vi "Manip5.vi"() -> ()   [LabVIEW 2021]
uses:
  <vilib>/numeric/Random Number (Range) U64.vi
  <vilib>/numeric/sub_Random U32.vi
panel:
  out "x > 7?":bool
  in  "Delay":u32
  out "Frequence":dbl
  out "Amplitude":dbl
  in  "stop":bool
  out "Waveform Chart":dynamicdata(graph)
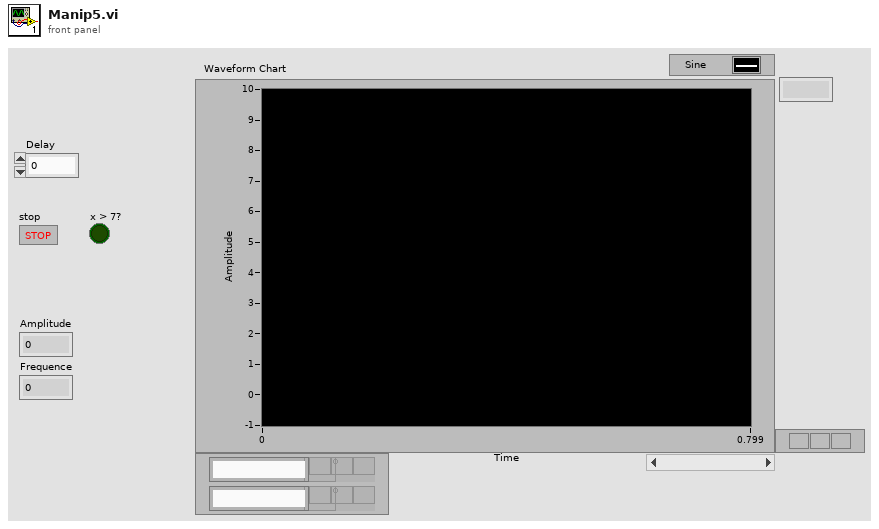
[diagram p1: front panel]
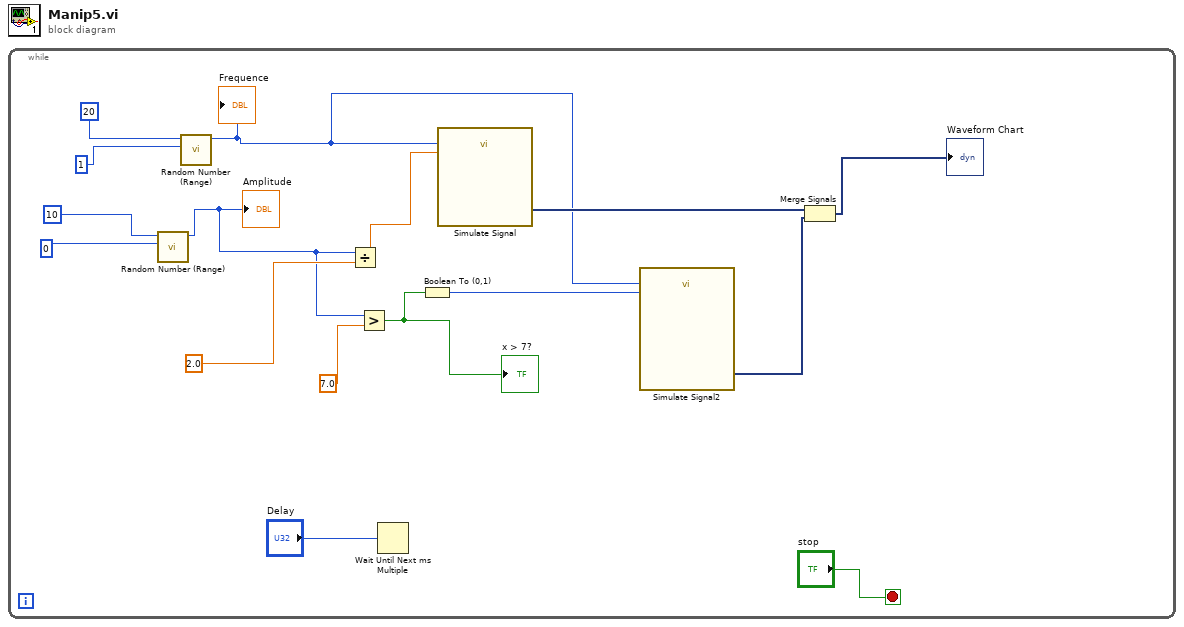
[diagram p0: block diagram]
diagram:
  n1 = while {
    stop <- "stop" stop-if-true
    n2 = call-poly <vilib>:"Random Number (Range).vi"("lower bound (0)"=u64 0 ("upper bound (100)"), "upper bound (100)"=u64 10) -> ("number"=w1:u64)  [unwired: 9 in]
    "Amplitude" <- w1
    n3 = call-poly <vilib>:"Random Number (Range).vi"("lower bound (0)"=u64 1 ("upper bound (100)"), "upper bound (100)"=u64 20) -> ("number"=w5:u64)  [unwired: 9 in]
    "Frequence" <- w5
    n4 = Divide(x=w1, y=2.0) -> (x/y=w2:dbl)
    n5 = Greater?(x=w1, y=7.0) -> (0:w7:bool)
    "x > 7?" <- w7
    n6 = Wait Until Next ms Multiple(millisecond multiple="Delay") -> ()  [unwired: 1 out]
    n7 = Boolean To (0,1)(Boolean=w7) -> (0, 1=w6:i16)
    n8 = call "Simulate Signal"("Frequency"=w5, "Amplitude"=w2) -> ("Sine"=w9:dynamicdata)  [unwired: 12 in, 1 out]
    n9 = call "Simulate Signal2"("Frequency"=w5, "Amplitude"=w6) -> ("Square"=w4:dynamicdata)  [unwired: 12 in, 1 out]
    n10 = Merge Signals(w9, w4) -> (→"Waveform Chart":dynamicdata)
  }
